vi "Ih_Image_FlipH.vi"(11 "2D array in":u32[][](array[numeric])) -> (3 "Flip H 2D array out":u32[][](array[numeric]))   [LabVIEW 2017]
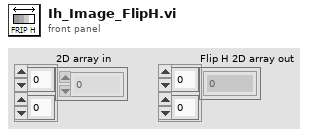
[diagram p1: front panel]
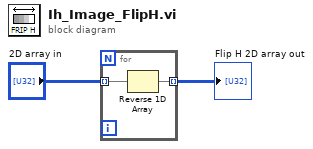
[diagram p0: block diagram]
diagram:
  n1 = for {
    tunnel: "2D array in" -> [w4] mode=indexing
    tunnel: [w3] -> w2 mode=indexing
    n2 = Reverse 1D Array(array=w4) -> (reversed array=w3:u32[])
  }
  "Flip H 2D array out" <- w2
